vi "RefWorkingFile.vi"() -> ()   [LabVIEW 2012, in "StimulCtrls.lvlib"]
uses:
  StimulCtrls.lvlib
panel:
  in  "Working File Refnum":refnum<file>
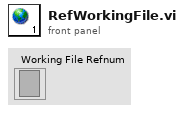
[diagram p1: front panel]
diagram:
